vi "Move_mm_Updated.vi"(8 "error in (no error)":errorcluster, 11 "Lifter_motor in":refnum<class "Lifter_motor.lvclass">) -> (0 "error out":errorcluster, 3 "Lifter_motor out":refnum<class "Lifter_motor.lvclass">)   [LabVIEW 2019, in "Lifter_motor.lvclass"]
uses:
  Lifter_motor.lvclass
  Lifter_motor.lvclass/Lifter_motor.ctl
  TCP Class/LifterTCP.lvclass
panel:
  in  "mm":dbl
  out "Driver ACK?":bool
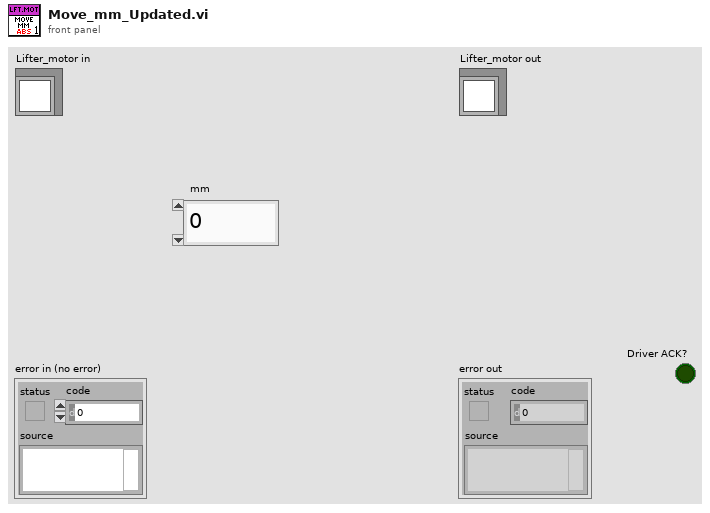
[diagram p1: front panel]
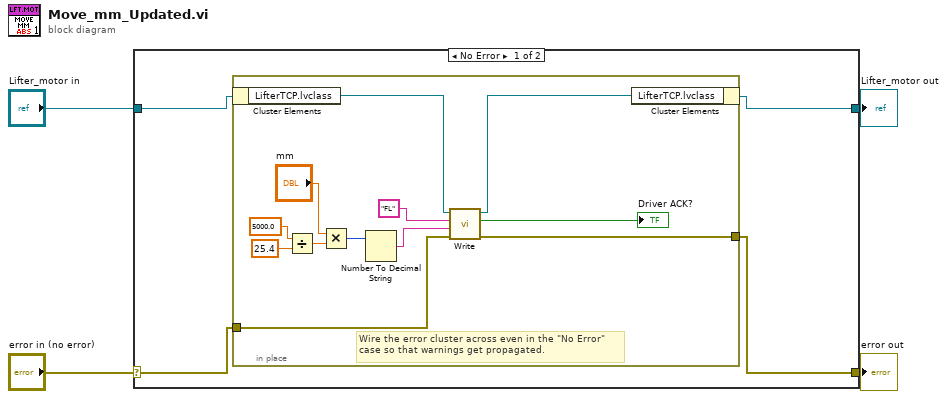
[diagram p0: block diagram]
diagram:
  n1 = case shown="No Error" "error in (no error)" {
    selector: "error in (no error)" -> [w5 w22]
    tunnel: [w8 w22] -> w3
    tunnel: [w7 w21] -> w1
    tunnel: "Lifter_motor in" -> [w6 w21]
    frame No Error {
      n2 = in-place {
        in-place-border: w5 -> [w12]
        in-place-border: [w11] -> w8
        # "Wire the error cluster across even in the \"No Error\"\ncase so that warnings get propagated."
        n3 = in-place-cluster #1(w6) -> ("LifterTCP.lvclass"=w13:refnum<class "LifterTCP.lvclass">)
        n4 = Divide(x=5000.0, y=25.4) -> (x/y=w19:dbl)
        n5 = Multiply(x="mm", y=w19) -> (x*y=w20:i32)
        n6 = Number To Decimal String(number=w20) -> (decimal integer string=w15:string)  [unwired: 1 in]
        n7 = call "Write.vi"("error in (no error)"=w12, "Parameter 2"=w15, "Parameter 1"="FL" ("string"), "LifterTCP in"=w13) -> ("error out"=w11:errorcluster, "Driver ACK?"=→"Driver ACK?":bool, "LifterTCP out"=w9:refnum<class "LifterTCP.lvclass">)  [unwired: 5 in]
        n8 = in-place-cluster #1("LifterTCP.lvclass"=w9) -> (w7:refnum<class "Lifter_motor.lvclass">)
      }
    }
    frame Error {
    }
  }
  "error out" <- w3
  "Lifter_motor out" <- w1
